vi "Save Load PID.vi"(7 "Name":string, 8 "error in":errorcluster, 10 "PID (in)":T1, 11 "Save Load Info (in)":T2) -> (0 "error out":errorcluster, 2 "PID (out)":T1, 3 "Save Load Info (out)":T2)   [LabVIEW 2016]
uses:
  Load Save Info.ctl
  <vilib>/Utility/config.llb/Config Data RefNum.ctl
  PID Settings.ctl
  <vilib>/Rock Robotics/Network Tables/NT Write Numeric Array.vi
  <vilib>/Utility/config.llb/Write Key (Double).vi
  <vilib>/Rock Robotics/Network Tables/NT Read Numeric Array.vi
  <vilib>/Utility/config.llb/Read Key (Double).vi
  <vilib>/Utility/config.llb/NI_LVConfig.lvlib
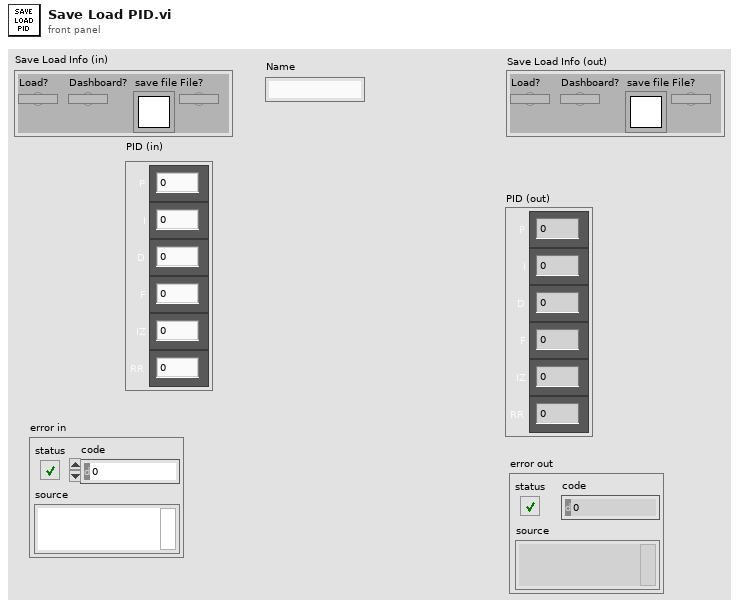
[diagram p1: front panel]
types:
  T1 = typedef "PID Settings.ctl" = cluster{"D":dbl, "F":dbl, "RR":dbl, "IZ":dbl, "P":dbl, "I":dbl}
  T2 = typedef "Load Save Info.ctl" = cluster{"Load?":bool, "Dashboard?":bool, "save file":T3, "File?":bool}
  T3 = typedef "NI_LVConfig.lvlib/Config Data RefNum.ctl" = refnum<k1>
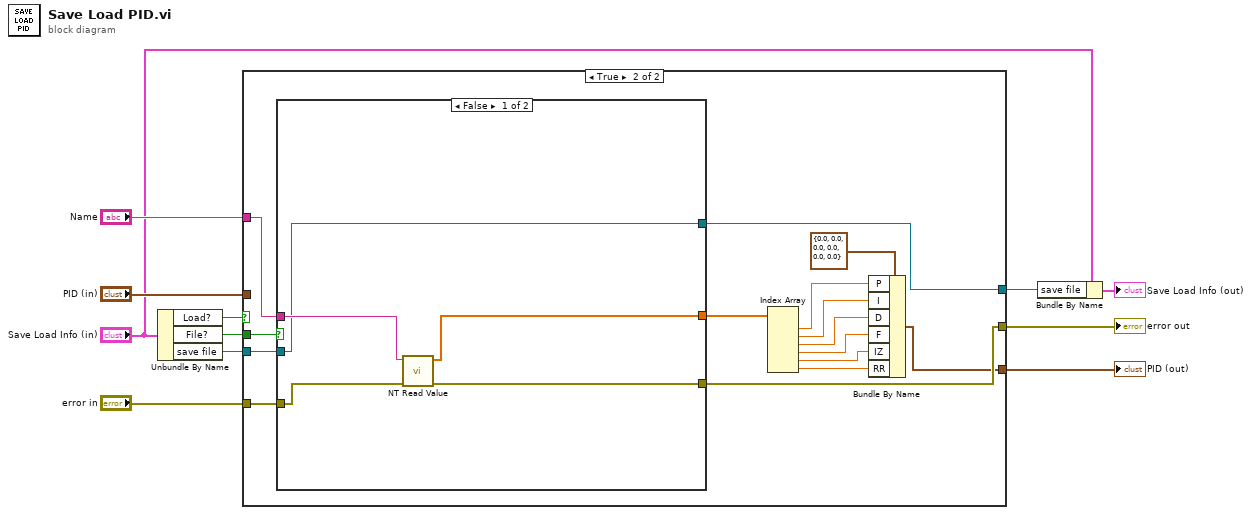
[diagram p0: block diagram]
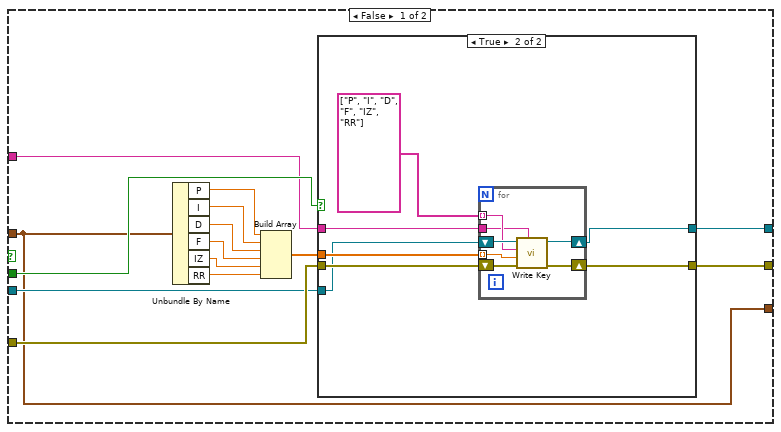
[diagram p2: hidden frame]
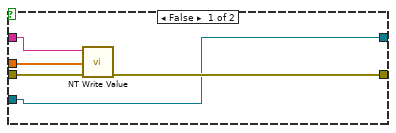
[diagram p3: hidden frame]
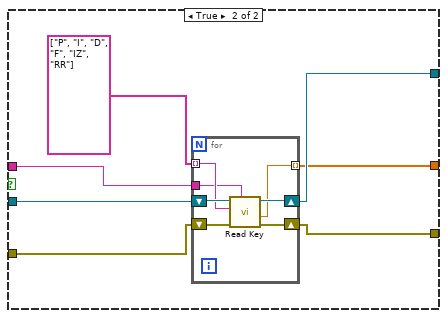
[diagram p4: hidden frame]
diagram:
  n1 = Unbundle By Name("Save Load Info (in)") -> ("Load?"=w11:bool, "File?"=w10:bool, "save file"=w6:T3)
  n2 = case shown="True" w11 {
    tunnel: w10 -> [w18 w59]
    tunnel: "Name" -> [w17 w49]
    tunnel: "PID (in)" -> [w12 _]
    tunnel: "error in" -> [w16 w51]
    tunnel: w6 -> [w15 w50]
    tunnel: [w14 w47] -> w5
    tunnel: [w13 w48] -> w2
    tunnel: [w12 w46] -> w1
    frame False {
      n3 = Unbundle By Name(w12) -> ("P"=w19:dbl, "I"=w20:dbl, "D"=w21:dbl, "F"=w22:dbl, "IZ"=w23:dbl, "RR"=w24:dbl)
      n4 = Build Array(w19, w20, w21, w22, w23, w24) -> (w25:dbl[])
      n5 = case shown="True" w18 {
        tunnel: w17 -> [w30 w36]
        tunnel: w25 -> [w29 w35]
        tunnel: w16 -> [w28 w37]
        tunnel: [w27 w33] -> w13
        tunnel: w15 -> [w26 w32]
        tunnel: [w26 w31] -> w14
        frame False {
          n6 = call-poly <vilib>:"NT Write Value.vi"("error in"=w28, "Numeric Array"=w29, "Name"=w30) -> ("error out"=w27:errorcluster)  [unwired: 8 in]
        }
        frame True {
          n7 = for {
            tunnel: w36 -> [w40]
            tunnel: string[] ["P", "I", "D", "F", "IZ", "RR"] -> [w41] mode=indexing
            shift-right: [w42] -> w33
            shift-left: w37 -> [w43]
            shift-right: [w39] -> w31
            shift-left: w32 -> [w44]
            tunnel: w35 -> [w38] mode=indexing
            n8 = call-poly <vilib>:"Write Key.vi"("section"=w40, "error in (no error)"=w43, "value"=w38, "key"=w41, "refnum"=w44) -> ("error out"=w42:errorcluster, "refnum out"=w39:T3)  [unwired: 4 in, 1 out]
          }
        }
      }
    }
    frame True {
      n9 = case shown="False" w59 {
        tunnel: w51 -> [w64 w71]
        tunnel: w50 -> [w60 w70]
        tunnel: w49 -> [w62 w68]
        tunnel: [w63 w67] -> w48
        tunnel: [w60 w66] -> w47
        tunnel: [w61 w65] -> w45
        frame False {
          n10 = call-poly <vilib>:"NT Read Value.vi"("error in"=w64, "Name"=w62) -> ("error out"=w63:errorcluster, "Numeric Array"=w61:dbl[])  [unwired: 8 in]
        }
        frame True {
          n11 = for {
            tunnel: w68 -> [w74]
            tunnel: string[] ["P", "I", "D", "F", "IZ", "RR"] -> [w75] mode=indexing
            shift-right: [w76] -> w67
            shift-left: w71 -> [w77]
            shift-right: [w73] -> w66
            shift-left: w70 -> [w78]
            tunnel: [w72] -> w65 mode=indexing
            n12 = call-poly <vilib>:"Read Key.vi"("section"=w74, "error in (no error)"=w77, "key"=w75, "refnum"=w78) -> ("error out"=w76:errorcluster, "value"=w72:dbl, "refnum out"=w73:T3)  [unwired: 4 in, 1 out]
          }
        }
      }
      n13 = Index Array(array=w45) -> (element #1=w53:dbl, element #2=w54:dbl, element #3=w55:dbl, element #4=w56:dbl, element #5=w57:dbl, element #6=w58:dbl)  [unwired: 6 in]
      n14 = Bundle By Name(cluster=T1 {"D"=0.0, "F"=0.0, "RR"=0.0, "IZ"=0.0, "P"=0.0, "I"=0.0} ("PID"), "P"=w53, "I"=w54, "D"=w55, "F"=w56, "IZ"=w57, "RR"=w58) -> (w46:T1)
    }
  }
  "error out" <- w2
  "PID (out)" <- w1
  n15 = Bundle By Name(cluster="Save Load Info (in)", "save file"=w5) -> (→"Save Load Info (out)":T2)
